vi "FirstDumper_Enable.vi"(0 "StopBool引用":refnum<vi>, 1 "SensorArray引用":refnum<vi>, 2 "Cmd":refnum<queue>, 3 "SolenNum_IN":refnum<queue>, 4 "SolenStatue_IN":refnum<queue>, 5 "错误输入（无错误）":errorcluster) -> (16 "Cmd_OUT":refnum<queue>, 17 "SolenNum_OUT":refnum<queue>, 18 "SolenStatue_OUT":refnum<queue>, 19 "错误输出":errorcluster)   [LabVIEW 2011]
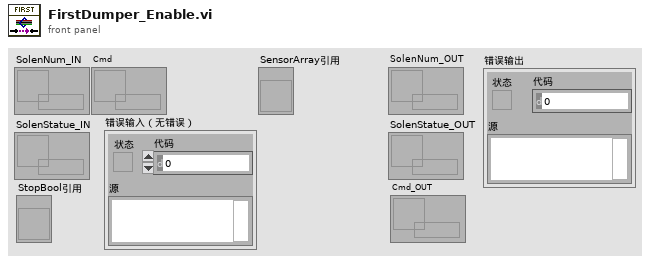
[diagram p1: front panel]
types:
  T1 = enum16{"None", "GetSensorStatue", "GetSensorAD", "GetSolenStatue", "GetPaltformStatue", "GetMotorStatue", "FeedMotorStart", "FeedMotorStop", "MotorStart", "MotorRestart", "MotorStop", "SolenAction", "SolenAdv", "RcvDataInit", "SetMotorSpeed", "Delay"}
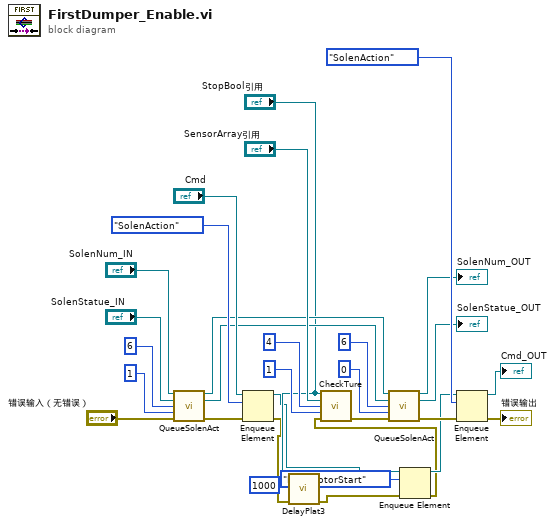
[diagram p0: block diagram]
diagram:
  n1 = call "QueueSolenAct.vi"("SolenNum_IN"="SolenNum_IN", "SolenStatue_IN"="SolenStatue_IN", "SolenNum_Value"=6, "SolenStatue_Value"=1, "错误输入（无错误）"="错误输入（无错误）") -> ("SolenNum_OUT"=w18:refnum<queue>, "SolenStatue_OUT"=w17:refnum<queue>, "错误输出"=w28:errorcluster)  [unwired: 8 in]
  n2 = Enqueue Element(queue="Cmd", element=T1."SolenAction" ("元素"), error in (no error)=w28) -> (queue out=w4:refnum<queue>, error out=w7:errorcluster)  [unwired: 1 in, 1 out]
  n3 = call "DelayPlat3.vi"("error In"=w7, "DelayTime"=u32 1000, "Bool"="StopBool引用") -> ("error Out"=w6:errorcluster)  [unwired: 8 in]
  n4 = Enqueue Element(queue=w4, element=T1."FeedMotorStart" ("元素"), error in (no error)=w6) -> (queue out=w3:refnum<queue>, error out=w1:errorcluster)  [unwired: 1 in, 1 out]
  n5 = call "CheckTure.vi"("Bool引用"="StopBool引用", "Array引用"="SensorArray引用", "索引"=4, "长度"=1, "错误输入（无错误）"=w1) -> ("错误输出"=w19:errorcluster)  [unwired: 10 in]
  n6 = call "QueueSolenAct.vi"("SolenNum_IN"=w18, "SolenStatue_IN"=w17, "SolenNum_Value"=6, "SolenStatue_Value"=0, "错误输入（无错误）"=w19) -> ("SolenNum_OUT"=→"SolenNum_OUT":refnum<queue>, "SolenStatue_OUT"=→"SolenStatue_OUT":refnum<queue>, "错误输出"=w14:errorcluster)  [unwired: 8 in]
  n7 = Enqueue Element(queue=w3, element=T1."SolenAction" ("元素"), error in (no error)=w14) -> (queue out=→"Cmd_OUT":refnum<queue>, error out=→"错误输出":errorcluster)  [unwired: 1 in, 1 out]
